vi "Test 2 Paths Cross in Past.vi"(8 "error in (no error)":errorcluster, 11 "Test Case In":refnum<class "Vector Test.lvclass">) -> (0 "error out":errorcluster, 3 "Test Case Out":refnum<class "Vector Test.lvclass">)   [LabVIEW 2021, in "Vector Test.lvclass"]
uses:
  Vector Test.lvclass
  C:/Program Files (x86)/National Instruments/LabVIEW 2021/vi.lib/Astemes/LUnit/Test Case.lvclass
  <vilib>/Astemes/LUnit/Test Case.lvclass/Test Case.ctl
  <vilib>/Astemes/LUnit/Append Pass Result.vi
  <vilib>/Astemes/LUnit/Append Fail Result.vi
  Vector Test.lvclass/Vector Test.ctl
  Vector/Vector.lvclass
  <vilib>/Astemes/LUnit/Test Case.lvclass
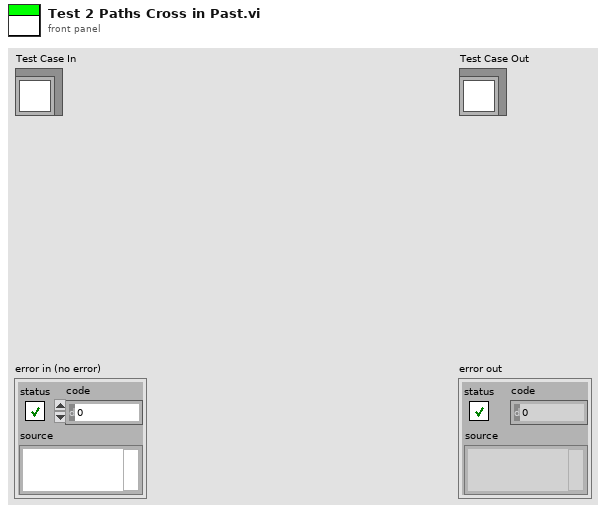
[diagram p1: front panel]
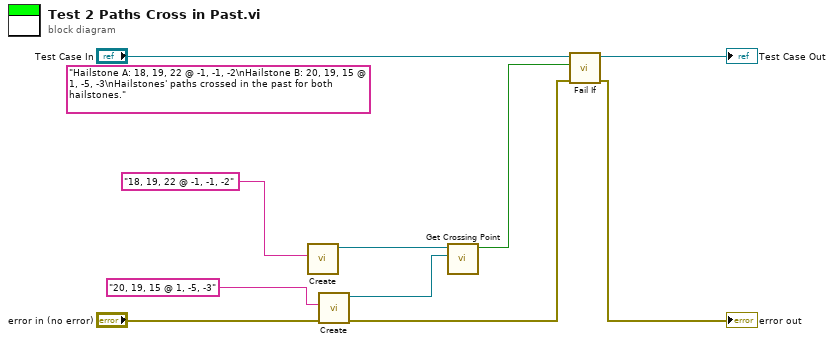
[diagram p0: block diagram]
diagram:
  (unwired) "Hailstone A: 18, 19, 22 @ -1, -1, -2\nHailstone B: 20, 19, 15 @ 1, -5, -3\nHailstones' paths crossed in the past for both hailstones." ("Input")
  n1 = call "Create.vi"("Input"="18, 19, 22 @ -1, -1, -2") -> ("Hailstone Out"=w3:refnum<class "Vector.lvclass">)  [unwired: 9 in, 1 out]
  n2 = call "Create.vi"("error in (no error)"="error in (no error)", "Input"="20, 19, 15 @ 1, -5, -3") -> ("error out"=w6:errorcluster, "Hailstone Out"=w2:refnum<class "Vector.lvclass">)  [unwired: 8 in]
  n3 = call "Get Crossing Point.vi"("Vector 2"=w2, "Vector in"=w3) -> ("In Future?"=w1:bool)  [unwired: 8 in, 1 out]
  n4 = call <vilib>:"Fail If.vi"("error in (no error)"=w6, "Fail?"=w1, "LUnit Test Case In"="Test Case In") -> ("error out"=→"error out":errorcluster, "LUnit Test Case Out"=→"Test Case Out":refnum<class "Vector Test.lvclass">)  [unwired: 7 in]
